vi "Destroy RTV.vi"(0 "RT Variables":refnum<class "RT Variables.lvclass">, 11 "error in (no error)":errorcluster) -> (4 "RT Variables":refnum<class "RT Variables.lvclass">, 15 "error out":errorcluster)   [LabVIEW 2019, in "LSL.lvlib" / "RT Variables.lvclass"]
uses:
  RT Variables.lvclass
  RT Variables.lvclass/RT Variables.ctl
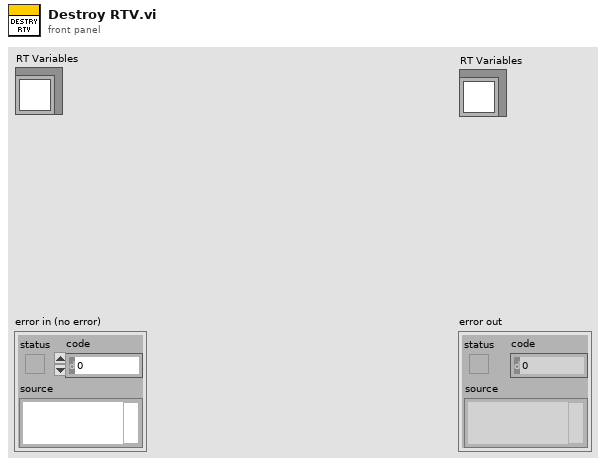
[diagram p1: front panel]
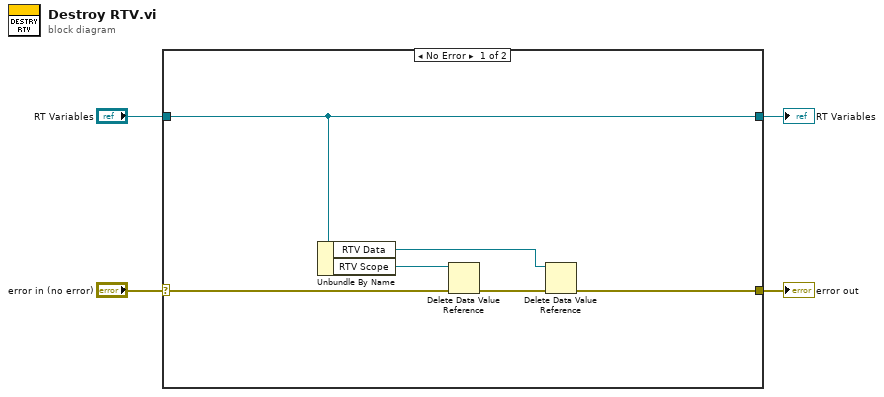
[diagram p0: block diagram]
diagram:
  n1 = case shown="No Error" "error in (no error)" {
    selector: "error in (no error)" -> [w10 w12]
    tunnel: [w6 w12] -> w3
    tunnel: [w9 w11] -> w2
    tunnel: "RT Variables" -> [w9 w11]
    frame No Error {
      n2 = Unbundle By Name(w9) -> ("RTV Data"=w5:refnum<data-value>, "RTV Scope"=w7:refnum<data-value>)
      n3 = Delete Data Value Reference(data value reference=w7, error in=w10) -> (error out=w8:errorcluster)  [unwired: 1 out]
      n4 = Delete Data Value Reference(data value reference=w5, error in=w8) -> (error out=w6:errorcluster)  [unwired: 1 out]
    }
    frame Error {
    }
  }
  "error out" <- w3
  "RT Variables" <- w2
